vi "AuMT8852B Error State Query.vi"(8 "error in (no error)":errorcluster, 11 "VISA session":refnum<visa-resource-name>) -> (0 "error out":errorcluster, 2 "error code":i32, 3 "VISA session out":refnum<visa-resource-name>, 4 "Results":T1)   [LabVIEW 2017]
doc: "Anritsu MT8852B Bluetooth Tester\n\nReturns information about recent errors and clears the error data from the instrument.\n\nOUTPUTS\nResults - error information:\nDUT HCI status - whether or not a DUT HCI error occurred.\nHCI error code - hexadecimal byte designating which error occurred.\nHCI error command - HCI command during which error occurred.\nSyntax error command - last GPIB command that caused a syntax error.\nExecution error command - last GPIB command that caused an execution error."
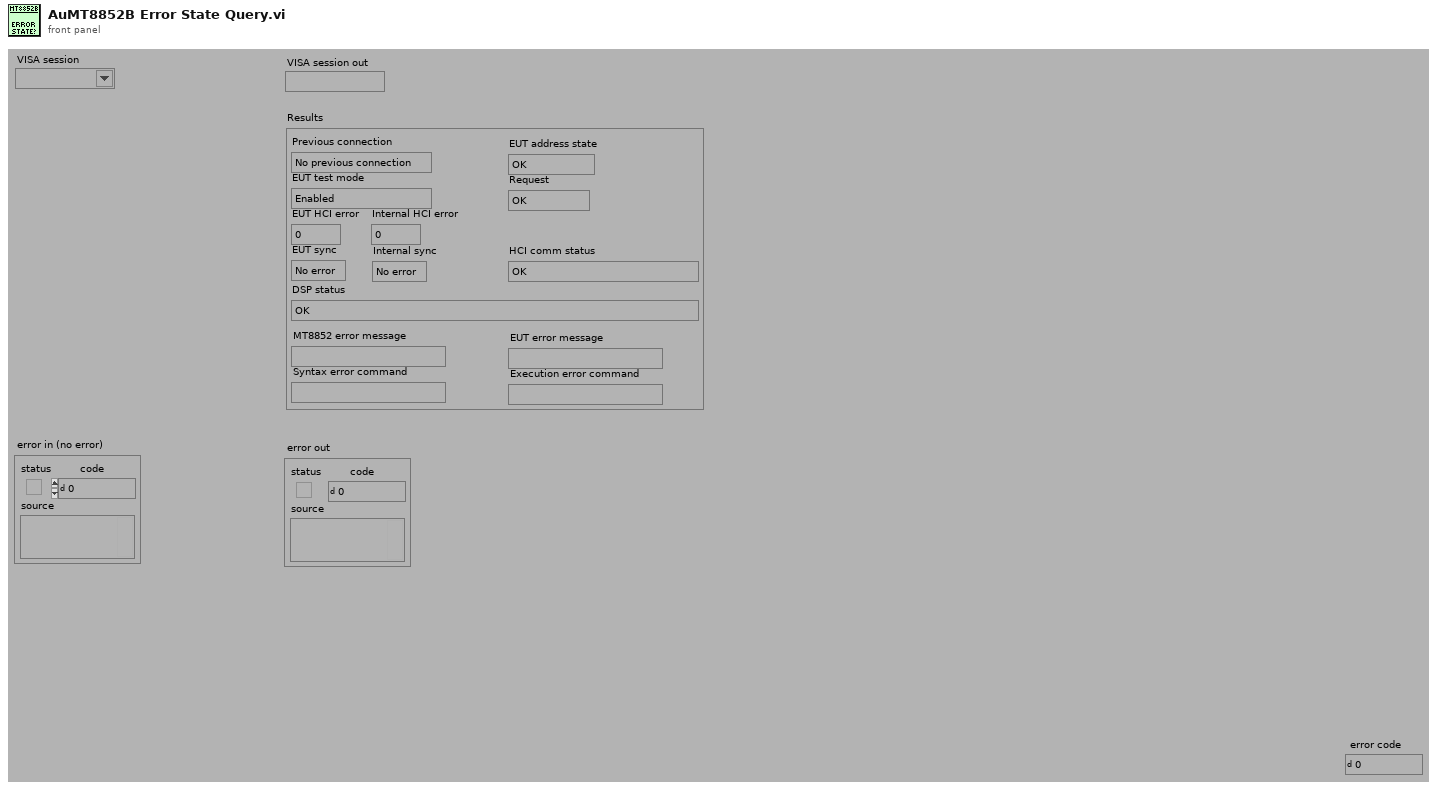
[diagram p1: front panel]
types:
  T1 = cluster{"MT8852 error message":string, "Syntax error command":string, "Execution error command":string, "EUT error message":string, "Previous connection":enum16{"No previous connection", "Previous connection"}, "EUT test mode":enum16{"Enabled", "Disabled"}, "EUT HCI error":i32, "Internal HCI error":i32, "EUT sync":enum16{"No error", "Error"}, "Internal sync":enum16{"No error", "Error"}, "Request":enum16{"OK", "Request failed"}, "EUT address state":enum16{"OK", "No address"}, "DSP status":enum16{"OK", "Searching channel", "Searching sync word", "Incorrect packet length", "No payload", "Auto ranging", "Incorrect packet", "Incorrect packet type", "Over range", "Under range", "Invalid payload", "Error finding start of packet using power profile", "Error locating GFSK sync word", "Location of GFSK sync word exceeds allowed limits", "Error locating EDR sync word", "Location of EDR sync word exceeds allowed limits", "Error decoding the packet type field", "Modulation mode of pi/4-DQPSK or 8DPSK not supported", "Specified (pi/4-DQPSK) modulation mode does not agree with detected packet type", "Specified (8DPSK) modulation mode does not agree with detected packet type", "Invalid packet type decoded", "Unknown packet type decoded", "Expected and measured packet lengths do not match", "Insufficient blocks in packet for measurement"}, "HCI comm status":enum16{"OK", "Unknown HCI command", "No connection", "Hardware failure", "Paging timeout", "Connection timeout", "Unsupported feature parameter", "Connection ended by user", "Low resource connection ended", "Power off connection ended", "Local host connection ended", "Unsupported remote feature", "Role change not allowed", "LMP response timeout", "IQ modem DAC saturation"}}
  T2 = enum16{"Simulate", "Range check", "Cache", "Query instrument status"}
  T3 = cluster{"MT8850 error message":string, "Syntax error command":string, "Execution error command":string, "EUT error message":string, "Previous connection":enum16{"No previous connection", "Previous connection"}, "EUT test mode":enum16{"Disabled", "Enabled"}, "EUT HCI error":i32, "Internal HCI error":i32, "EUT sync":enum16{"No error", "Error"}, "Internal sync":enum16{"No error", "Error"}, "Request":enum16{"OK", "Request failed"}, "EUT address state":enum16{"OK", "No address"}, "DSP status":enum16{"OK", "Searching channel", "Searching sync word", "Incorrect packet length", "No payload", "Auto ranging", "Incorrect packet", "Incorrect packet type", "Over range", "Under range", "Invalid payload"}, "HCI comm status":enum16{"OK", "Unknown HCI command", "No connection", "Hardware failure", "Paging timeout", "Connection timeout", "Unsupported feature parameter", "Connection ended by user", "Low resource connection ended", "Power off connection ended", "Local host connection ended", "Unsupported remote feature", "Role change not allowed", "LMP response timeout"}}
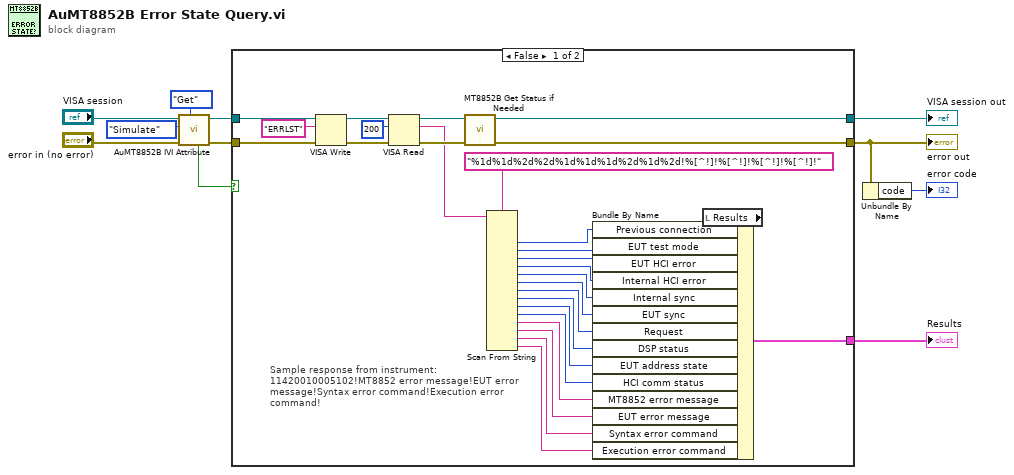
[diagram p0: block diagram]
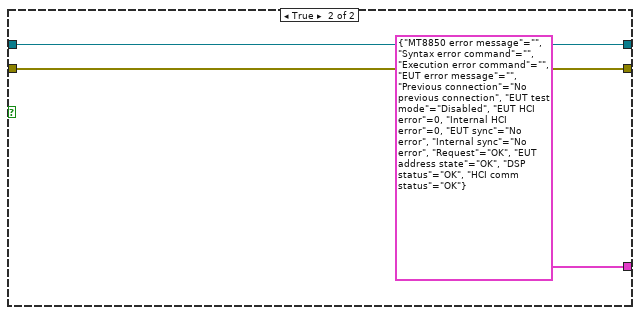
[diagram p2: hidden frame]
diagram:
  n1 = call <instrlib>:"AuMT8852B IVI Attribute.vi"("Set/Get (Set)"=enum16{"Set", "Get"}."Get", "error in (no error)"="error in (no error)", "Flag (Simulate)"=T2."Simulate", "VISA session"="VISA session") -> ("error out"=w7:errorcluster, "VISA session out"=w8:refnum<visa-resource-name>, "Value out"=w4:bool)  [unwired: 5 in]
  n2 = case shown="False" w4 {
    tunnel: [w36 w41] -> w1
    tunnel: [w37 w42] -> w9
    tunnel: w8 -> [w39 w42]
    tunnel: w7 -> [w38 w41]
    tunnel: [w28 T3 {"MT8850 error message"="", "Syntax error command"="", "Execution error command"="", "EUT error message"="", "Previous connection"=enum."No previous connection", "EUT test mode"=enum."Disabled", "EUT HCI error"=0, "Internal HCI error"=0, "EUT sync"=enum."No error", "Internal sync"=enum."No error", "Request"=enum."OK", "EUT address state"=enum."OK", "DSP status"=enum."OK", "HCI comm status"=enum."OK"} ("Results")] -> w2
    frame False {
      # "Sample response from instrument:\n11420010005102!MT8852 error message!EUT error message!Syntax error command!Execution error command!"
      n3 = VISA Write(VISA resource name=w39, write buffer="ERRLST" ("write buffer (\"\")"), error in (no error)=w38) -> (VISA resource name out=w35:refnum<visa-resource-name>, error out=w32:errorcluster)  [unwired: 1 out]
      n4 = VISA Read(VISA resource name=w35, byte count=u32 200 ("byte count (0)"), error in (no error)=w32) -> (VISA resource name out=w31:refnum<visa-resource-name>, read buffer=w27:string, error out=w30:errorcluster)  [unwired: 1 out]
      n5 = call <instrlib>:"MT8852B Get Status if Needed.vi"("error in (no error)"=w30, "VISA session"=w31) -> ("error out"=w36:errorcluster, "VISA session out"=w37:refnum<visa-resource-name>)  [unwired: 8 in]
      n6 = Scan From String(format string="%1d%1d%2d%2d%1d%1d%1d%2d%1d%2d!%[^!]!%[^!]!%[^!]!%[^!]!", input string=w27) -> (output 1=w26:i32, output 2=w25:i32, output 3=w24:i32, output 4=w23:i32, output 5=w22:i32, output 6=w21:i32, output 7=w20:i32, output 8=w19:i32, output 9=w18:i32, output 10=w17:i32, output 11=w15:string, output 12=w14:string, output 13=w13:string, output 14=w12:string)  [unwired: 16 in, 3 out]
      n7 = local read "Results"() -> (w29:T1)
      n8 = Bundle By Name(cluster=w29, "Previous connection"=w26, "EUT test mode"=w25, "EUT HCI error"=w24, "Internal HCI error"=w23, "Internal sync"=w22, "EUT sync"=w21, "Request"=w20, "DSP status"=w19, "EUT address state"=w18, "HCI comm status"=w17, "MT8852 error message"=w15, "EUT error message"=w14, "Syntax error command"=w13, "Execution error command"=w12) -> (w28:T1)
    }
    frame True {
    }
  }
  "error out" <- w1
  "VISA session out" <- w9
  "Results" <- w2
  n9 = Unbundle By Name(w1) -> ("code"=→"error code":i32)
